vi "海流计设置窗口.vi"() -> (2 "开关":bool, 3 "确定输出":bool)   [LabVIEW 2016, in "AADI5400.lvlib"]
uses:
  AADI5400.lvlib
  <vilib>/Instr/_visa.llb/VISA Configure Serial Port (Instr).vi
  <vilib>/ptbypt/NI_PtbyPt.lvlib
  <vilib>/Utility/config.llb/NI_LVConfig.lvlib
panel:
  in  "波特率":u32=115200
  in  "流控制":u16(ring) items=["None", "XON/XOFF", "RTS/CTS", "XON/XOFF & RTS/CTS", "DTR/DSR", "XON/XOFF & DTR/DSR"]
  in  "海流计序列号":string
  out "串口开关状态":bool
  in  "海流计型号":string(combo)="DCPS 5400"
  in  "字符串":string
  in  "串口":refnum<visa-resource-name>="COM6"
  in  "确定":bool
  in  "取消":bool
  in  "串口开关":bool
  # "剖面海流计参数"
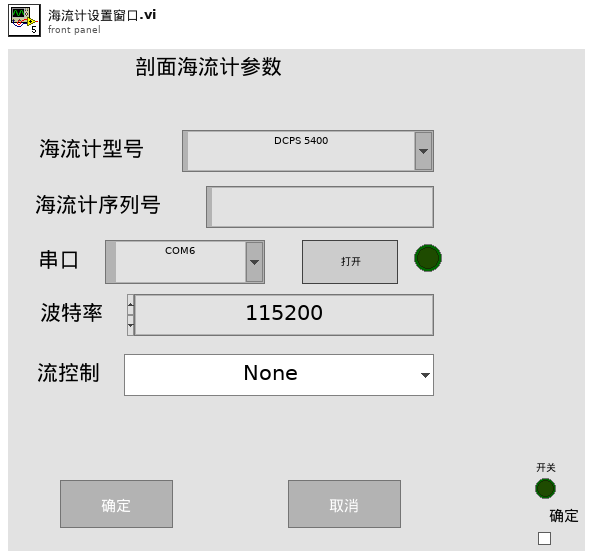
[diagram p1: front panel]
types:
  T1 = enum8{"Enabled", "Disabled", "Disabled and Grayed Out"}
  T2 = typedef "NI_LVConfig.lvlib/Config Data RefNum.ctl" = refnum<k1>
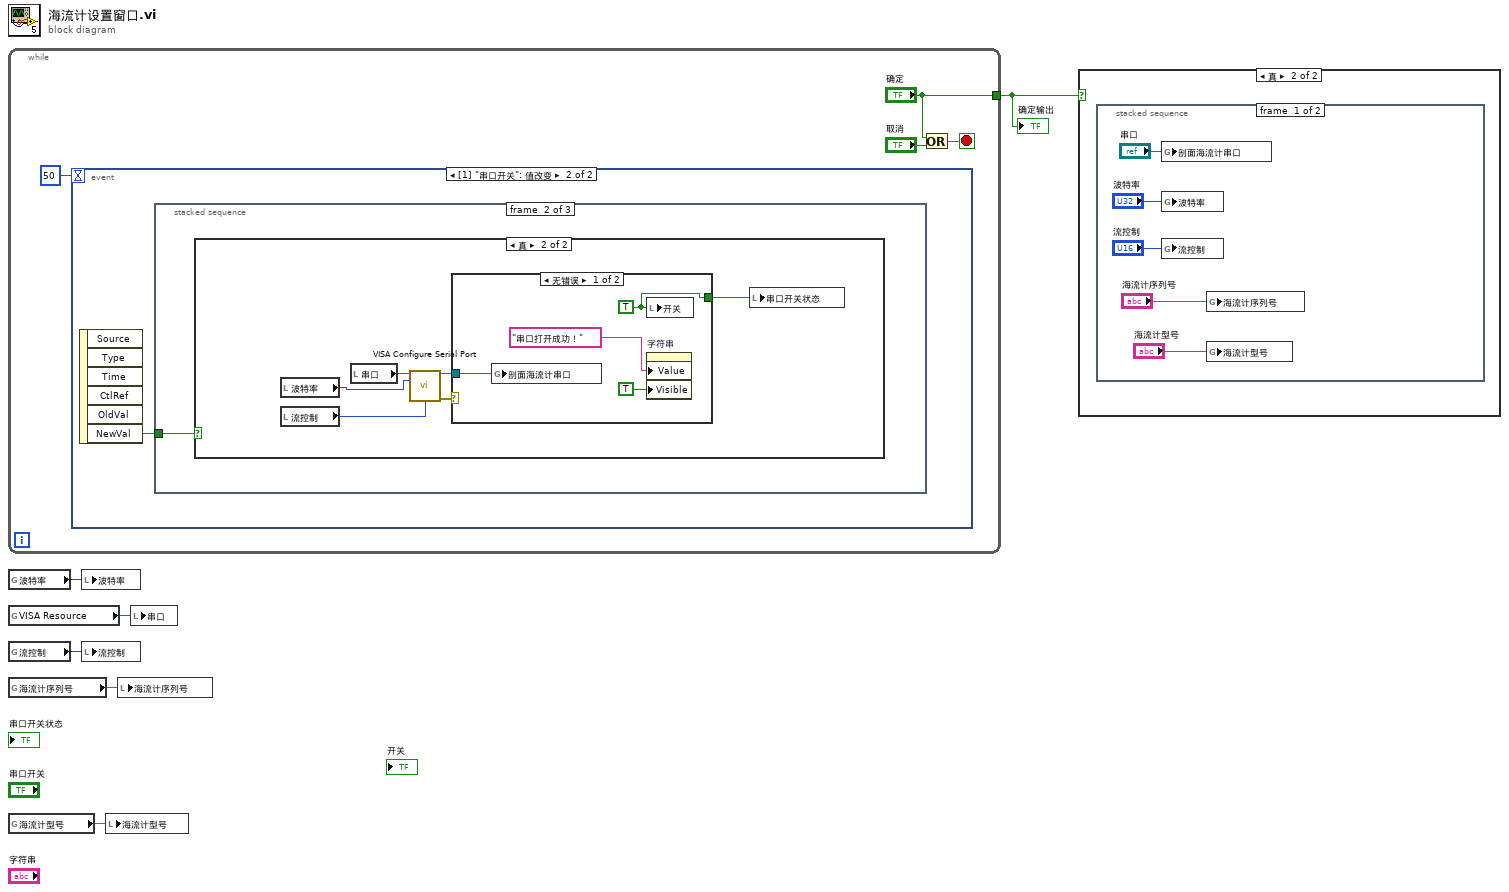
[diagram p0: block diagram]
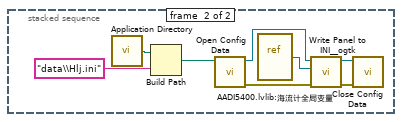
[diagram p3: hidden frame]
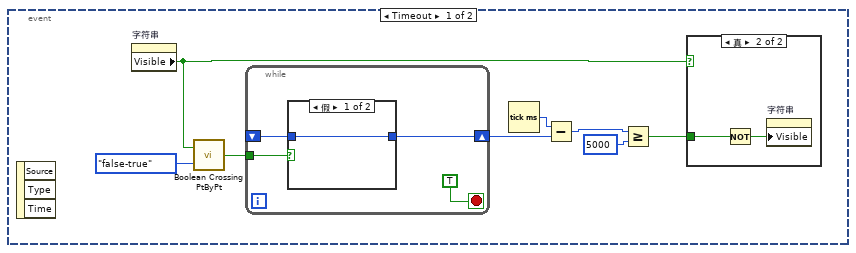
[diagram p4: hidden frame]
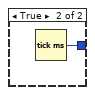
[diagram p6: hidden frame]
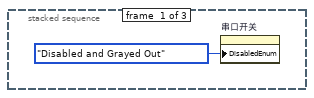
[diagram p7: hidden frame]
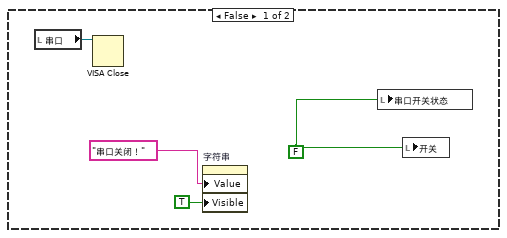
[diagram p8: hidden frame]
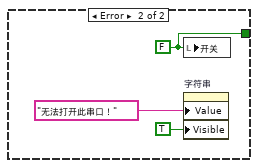
[diagram p9: hidden frame]
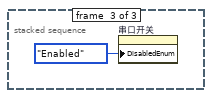
[diagram p10: hidden frame]
diagram:
  n1 = while {
    tunnel: ["确定"] -> w5
    stop <- w8 stop-if-true
    n2 = event shown="[1] \"串口开关\": 值改变" {
      selector: _ -> [_ _]
      dyn-events: _ -> [_ _]
      timeout: 50 -> [_ _]
      event Timeout {
        n3 = event-data() -> ()  [unwired: 1 in, 3 out]
        n4 = property on="字符串" class="Str"() -> ("Visible"=w12:bool)  [unwired: 2 in, 2 out]
        n5 = call <vilib>:"Boolean Crossing PtByPt.vi"("direction"=enum16{"either", "false-true", "true-false"}."false-true", "input"=w12) -> ("crossing"=w17:bool)  [unwired: 1 in]
        n6 = while {
          tunnel: w17 -> [w24]
          shift-right: [w22] -> w15
          shift-left: _ -> [w21]
          stop <- TRUE stop-if-true
          n7 = case shown="假" w24 {
            tunnel: [w25 w26] -> w22
            tunnel: w21 -> [w25 _]
            frame False {
            }
            frame True {
              n8 = Tick Count (ms)() -> (millisecond timer value=w26:u32)
            }
          }
        }
        n9 = Tick Count (ms)() -> (millisecond timer value=w16:u32)
        n10 = Subtract(x=w16, y=w15) -> (x-y=w14:u32)
        n11 = Greater Or Equal?(x=w14, y=u32 5000) -> (x >= y?=w11:bool)
        n12 = case shown="真" w12 {
          tunnel: w11 -> [_ w19]
          frame False {
          }
          frame True {
            n13 = Not(x=w19) -> (.not. x?=w20:bool)
            n14 = property on="字符串" class="Str"("Visible"=w20) -> ()  [unwired: 2 in, 2 out]
          }
        }
      }
      event "串口开关": Value Change {
        n15 = event-data() -> ("NewVal"=w27:bool)  [unwired: 1 in, 5 out]
        n16 = stacked-sequence {
          tunnel: w27 -> [_ w29 _]
          frame #0 {
            n17 = property on="串口开关" class="Bool"("DisabledEnum"=T1."Disabled and Grayed Out" ("禁用")) -> ()  [unwired: 2 in, 2 out]
          }
          frame #1 {
            n18 = case shown="真" w29 {
              frame False {
                w32 = FALSE
                n19 = local read "串口"() -> (w33:refnum<visa-resource-name>)
                n20 = VISA Close(VISA resource name=w33) -> ()  [unwired: 1 in, 1 out]
                n21 = property on="字符串" class="Str"("Value"="串口关闭！" ("字符串"), "Visible"=TRUE ("可见")) -> ()  [unwired: 2 in, 2 out]
                n22 = local write "串口开关状态"(w32) -> ()
                n23 = local write "开关"(w32) -> ()
              }
              frame True {
                n24 = local read "波特率"() -> (w38:u32)
                n25 = local read "流控制"() -> (w37:u16)
                n26 = local read "串口"() -> (w39:refnum<visa-resource-name>)
                n27 = call-poly "VISA Configure Serial Port"("VISA resource name"=w39, "baud rate (9600)"=w38, "flow control (0:none)"=w37) -> ("VISA resource name out"=w34:refnum<visa-resource-name>, "error out"=w36:errorcluster)  [unwired: 11 in]
                n28 = case shown="无错误" w36 {
                  tunnel: [w43 w44] -> w35
                  tunnel: w34 -> [w40 _]
                  frame No Error {
                    w43 = TRUE ("串口开关状态")
                    n29 = global write "海流计全局变量.vi" "剖面海流计串口"(w40) -> ()
                    n30 = local write "开关"(w43) -> ()
                    n31 = property on="字符串" class="Str"("Value"="串口打开成功！" ("字符串"), "Visible"=TRUE ("可见")) -> ()  [unwired: 2 in, 2 out]
                  }
                  frame Error {
                    w44 = FALSE ("串口开关状态")
                    n32 = local write "开关"(w44) -> ()
                    n33 = property on="字符串" class="Str"("Value"="无法打开此串口！" ("字符串"), "Visible"=TRUE ("可见")) -> ()  [unwired: 2 in, 2 out]
                  }
                }
                n34 = local write "串口开关状态"(w35) -> ()
              }
            }
          }
          frame #2 {
            n35 = property on="串口开关" class="Bool"("DisabledEnum"=T1."Enabled" ("禁用")) -> ()  [unwired: 2 in, 2 out]
          }
        }
      }
    }
    n36 = Or(x="确定", y="取消") -> (x .or. y?=w8:bool)
  }
  "确定输出" <- w5
  n37 = global read "海流计全局变量.vi" "波特率"() -> (w2:u32)
  n38 = global read "全局_综合生物毒性.vi" "VISA Resource"() -> (w6:refnum<visa-resource-name>)
  n39 = global read "海流计全局变量.vi" "流控制"() -> (w1:u16)
  n40 = global read "海流计全局变量.vi" "海流计序列号"() -> (w4:string)
  n41 = global read "海流计全局变量.vi" "海流计型号"() -> (w3:string)
  n42 = local write "波特率"(w2) -> ()
  n43 = local write "流控制"(w1) -> ()
  n44 = local write "海流计型号"(w3) -> ()
  n45 = local write "海流计序列号"(w4) -> ()
  n46 = local write "串口"(w6) -> ()
  n47 = case shown="真" w5 {
    frame False {
    }
    frame True {
      n48 = stacked-sequence {
        frame #0 {
          n49 = global write "海流计全局变量.vi" "剖面海流计串口"("串口") -> ()
          n50 = global write "海流计全局变量.vi" "波特率"("波特率") -> ()
          n51 = global write "海流计全局变量.vi" "流控制"("流控制") -> ()
          n52 = global write "海流计全局变量.vi" "海流计序列号"("海流计序列号") -> ()
          n53 = global write "海流计全局变量.vi" "海流计型号"("海流计型号") -> ()
        }
        frame #1 {
          n54 = call <vilib>:"Application Directory.vi"() -> ("Application Directory"=w56:path)
          n55 = Build Path(base path=w56, name or relative path="data\\Hlj.ini" ("名称或相对路径")) -> (appended path=w58:path)
          n56 = call <vilib>:"Open Config Data.vi"("configuration file path"=w58) -> ("error out"=w54:errorcluster, "refnum"=w59:T2)  [unwired: 8 in, 1 out]
          n57 = vi-ref "AADI5400.lvlib:海流计全局变量.vi"() -> (w53:refnum<vi>)
          n58 = call <userlib>:"Write Panel to INI__ogtk.vi"("error in (no error)"=w54, "VI ref"=w53, "refnum"=w59) -> ("error out"=w55:errorcluster, "refnum out"=w60:T2)  [unwired: 7 in]
          n59 = call <vilib>:"Close Config Data.vi"("error in (no error)"=w55, "refnum"=w60) -> ()  [unwired: 8 in, 2 out]
        }
      }
    }
  }
